vi "Stack.vi"(2 "Array":u16[](array[numeric])) -> (10 "Min":u16, 11 "Max":u16, 14 "appended array":u16[](array[numeric]), 15 "appended array 2":u16[](array[numeric]), 16 "appended array 3":u16[](array[numeric]), 17 "appended array 4":u16[](array[numeric]), 18 "appended array 5":u16[](array[numeric]), 19 "appended array 6":u16[](array[numeric]))   [LabVIEW 2017]
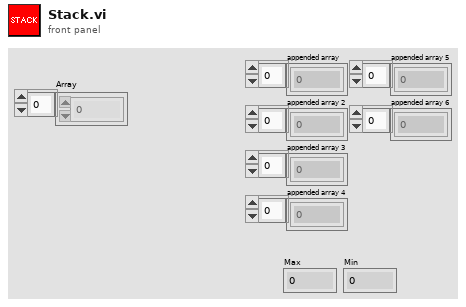
[diagram p1: front panel]
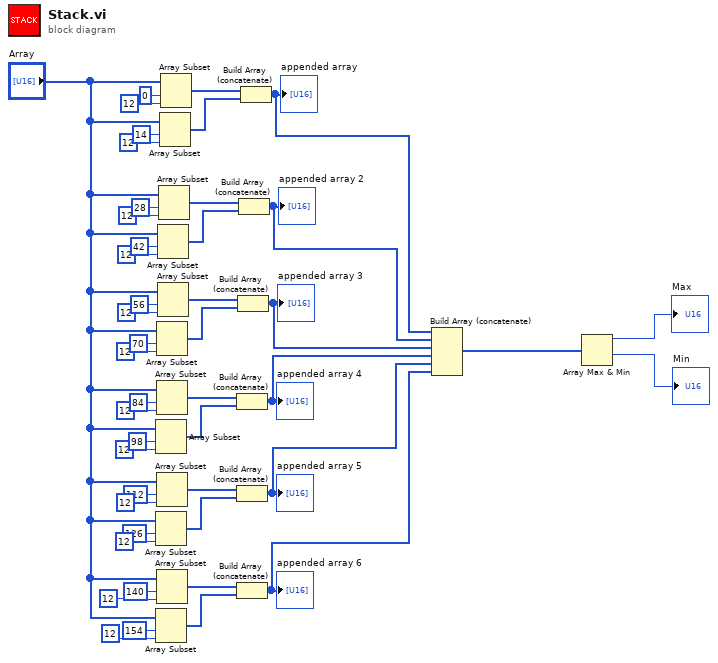
[diagram p0: block diagram]
diagram:
  n1 = Array Subset(array="Array", index=98, length=12) -> (w23:u16[])
  n2 = Array Subset(array="Array", index=126, length=12) -> (w17:u16[])
  n3 = Array Subset(array="Array", index=154, length=12) -> (w11:u16[])
  n4 = Array Subset(array="Array", index=70, length=12) -> (w29:u16[])
  n5 = Array Subset(array="Array", index=84, length=12) -> (w28:u16[])
  n6 = Array Subset(array="Array", index=112, length=12) -> (w22:u16[])
  n7 = Array Subset(array="Array", index=140, length=12) -> (w16:u16[])
  n8 = Array Subset(array="Array", index=42, length=12) -> (w35:u16[])
  n9 = Array Subset(array="Array", index=56, length=12) -> (w34:u16[])
  n10 = Array Subset(array="Array", index=28, length=12) -> (w40:u16[])
  n11 = Array Subset(array="Array", index=14, length=12) -> (w41:u16[])
  n12 = Array Subset(array="Array", index=0, length=12) -> (w46:u16[])
  n13 = Build Array (concatenate)(w28, w23) -> (w6:u16[])
  "appended array 4" <- w6
  n14 = Build Array (concatenate)(w22, w17) -> (w5:u16[])
  "appended array 5" <- w5
  n15 = Build Array (concatenate)(w16, w11) -> (w4:u16[])
  "appended array 6" <- w4
  n16 = Build Array (concatenate)(w34, w29) -> (w7:u16[])
  "appended array 3" <- w7
  n17 = Build Array (concatenate)(w40, w35) -> (w8:u16[])
  "appended array 2" <- w8
  n18 = Build Array (concatenate)(w46, w41) -> (w9:u16[])
  "appended array" <- w9
  n19 = Build Array (concatenate)(w9, w8, w7, w6, w5, w4) -> (w1:u16[])
  n20 = Array Max & Min(array=w1) -> (max value=→"Max":u16, min value=→"Min":u16)  [unwired: 2 out]
